vi "write_ini_file.vi"   [LabVIEW 2021]
uses:
  <vilib>/Utility/config.llb/Write Key (Boolean).vi
  <vilib>/Utility/config.llb/Write Key (Double).vi
  <vilib>/Utility/config.llb/Write Key (Path).vi
  <vilib>/Utility/config.llb/Write Key (String).vi
  <vilib>/Utility/config.llb/NI_LVConfig.lvlib
types:
  T1 = typedef "NI_LVConfig.lvlib/Config Data RefNum.ctl" = refnum<k1>
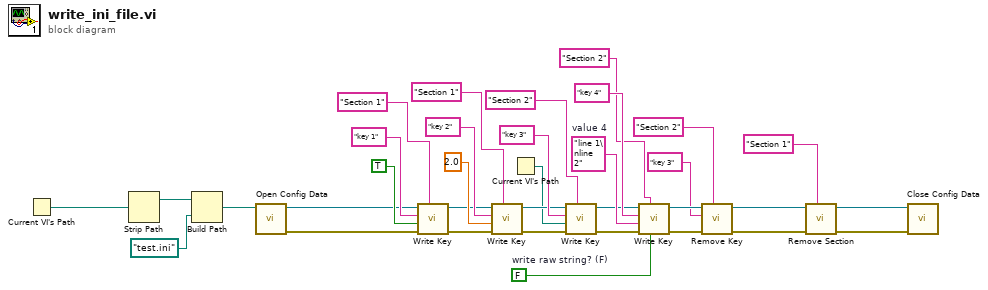
[diagram p0: block diagram]
diagram:
  w2 = FALSE  # write raw string? (F)
  w31 = "line 1\nline 2"  # value 4
  n1 = Current VI's Path() -> (path=w18:path)
  n2 = Strip Path(path=w18) -> (stripped path=w17:path)  [unwired: 1 out]
  n3 = Build Path(base path=w17, name or relative path=path "test.ini" ("default name")) -> (appended path=w1:path)
  n4 = call <vilib>:"Open Config Data.vi"("configuration file path"=w1) -> ("error out"=w23:errorcluster, "refnum"=w19:T1)  [unwired: 2 in, 7 out]
  n5 = call-poly <vilib>:"Write Key.vi"("section"="Section 1", "error in (no error)"=w23, "value"=TRUE ("value 1"), "key"="key 1" ("Key 1"), "refnum"=w19) -> ("error out"=w24:errorcluster, "refnum out"=w20:T1)  [unwired: 5 out]
  n6 = call-poly <vilib>:"Write Key.vi"("section"="Section 1", "error in (no error)"=w24, "value"=2.0 ("value 2"), "key"="key 2" ("Key 2"), "refnum"=w20) -> ("error out"=w25:errorcluster, "refnum out"=w21:T1)  [unwired: 3 in, 2 out]
  n7 = Current VI's Path() -> (path=w8:path)
  n8 = call-poly <vilib>:"Write Key.vi"("section"="Section 2", "error in (no error)"=w25, "value"=w8, "key"="key 3" ("Key 3"), "refnum"=w21) -> ("error out"=w26:errorcluster, "refnum out"=w22:T1)  [unwired: 5 out]
  n9 = call-poly <vilib>:"Write Key.vi"("write raw string? (F)"=w2, "section"="Section 2", "error in (no error)"=w26, "value"=w31, "key"="key 4" ("Key 4"), "refnum"=w22) -> ("error out"=w6:errorcluster, "refnum out"=w7:T1)  [unwired: 4 out]
  n10 = call <vilib>:"Remove Key.vi"("section"="Section 2", "error in (no error)"=w6, "key"="key 3", "refnum"=w7) -> ("error out"=w12:errorcluster, "refnum out"=w11:T1)  [unwired: 5 in, 1 out]
  n11 = call <vilib>:"Remove Section.vi"("section"="Section 1", "error in (no error)"=w12, "refnum"=w11) -> ("error out"=w9:errorcluster, "refnum out"=w10:T1)  [unwired: 6 in, 1 out]
  n12 = call <vilib>:"Close Config Data.vi"("error in (no error)"=w9, "refnum"=w10) -> ()  [unwired: 1 in, 9 out]
